vi "Delete Item.vi"(3 "Error in":errorcluster, 5 "Item":u32) -> (0 "Error out":errorcluster)   [LabVIEW 2020]
uses:
  <vilib>/Utility/config.llb/NI_LVConfig.lvlib
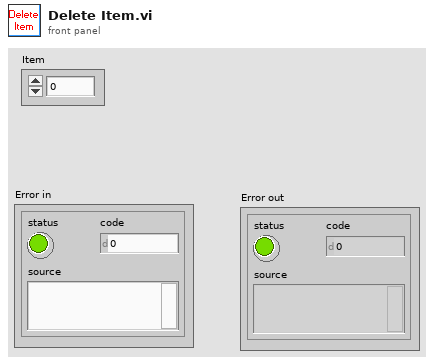
[diagram p1: front panel]
types:
  T1 = typedef "NI_LVConfig.lvlib/Config Data RefNum.ctl" = refnum<k1>
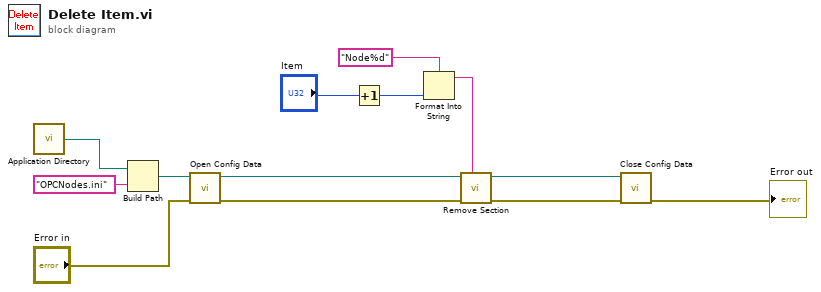
[diagram p0: block diagram]
diagram:
  n1 = call <vilib>:"Application Directory.vi"() -> ("Application Directory"=w13:path)
  n2 = Build Path(base path=w13, name or relative path="OPCNodes.ini") -> (appended path=w11:path)
  n3 = call <vilib>:"Open Config Data.vi"("error in (no error)"="Error in", "configuration file path"=w11) -> ("error out"=w5:errorcluster, "refnum"=w6:T1)  [unwired: 7 in, 1 out]
  n4 = Increment(x="Item") -> (x+1=w9:u32)
  n5 = Format Into String(format string="Node%d" ("section"), w9) -> (resulting string=w7:string)  [unwired: 2 in, 1 out]
  n6 = call <vilib>:"Remove Section.vi"("section"=w7, "error in (no error)"=w5, "refnum"=w6) -> ("error out"=w3:errorcluster, "refnum out"=w1:T1)  [unwired: 6 in, 1 out]
  n7 = call <vilib>:"Close Config Data.vi"("error in (no error)"=w3, "refnum"=w1) -> ("error out"=→"Error out":errorcluster)  [unwired: 8 in, 1 out]
